vi "File Page - Update Multi-Trig Controls.vi"(7 "File Ctl Refs in":T2, 8 "error in (no error)":errorcluster, 11 "Item Ref in":T1 format="%.0x") -> (0 "error out":errorcluster)   [LabVIEW 2015, in "Waveform Data Logger System Explorer.lvlib"]
uses:
  Waveform Data Logger System Explorer.lvlib
  Types/File Ctl Refs.ctl
  Types/File - Spec Ctl Refs.ctl
  Types/File - Wfm Ctl Refs.ctl
  Types/File - Settings Ctl Refs.ctl
  Shared/Classes/Log File Specifications/Log File Specification/File Conflict Operation.ctl
  Types/File - Start Trig Ctl Refs.ctl
  Shared/Types/Start Trigger.ctl
  Shared/Types/Default Trigger.ctl
  Shared/Types/Digital Trigger.ctl
  Shared/Types/Analog Trigger.ctl
  Shared/Types/In Range Trigger.ctl
  Shared/Types/Value Change Trigger.ctl
  Shared/Types/Boolean Trigger.ctl
  Types/Single Node Browser Data.ctl
  <vilib>/NI Veristand/UI Controls/Single Node Browser/Single Node Browser Ref.ctl
  NationalInstruments.VeriStand.SystemStorageUI
  <vilib>/NI Veristand/UI Controls/Single Node Browser/Callback Type.ctl
  <vilib>/NI Veristand/UI Controls/Single Node Browser/Net Event Data.ctl
  <vilib>/NI Veristand/UI Controls/Single Node Browser/Net Event.ctl
  Types/File - Stop Trig Ctl Refs.ctl
  Shared/Types/Stop Trigger.ctl
  Types/File - Advanced Ctl Refs.ctl
  Types/Log Timestamps.ctl
  <vilib>/NI Veristand/Custom Device API/Custom Device Item Ref.ctl
  Shared/Globals/Property Strings.vi
  <vilib>/NI Veristand/Custom Device API/Get Item Property (U16).vi
  <vilib>/NI Veristand/Custom Device API/Set Item Property (Boolean).vi
  <vilib>/NI Veristand/Custom Device API/Get Item Property (Boolean).vi
  Shared/Waveform Data Logger Shared.lvlib
  <vilib>/NI VeriStand/Custom Device API/Custom Device API.lvlib
  Shared/Classes/Log File Specifications/Log File Specification/Log File Specification.lvclass
  <vilib>/NI VeriStand/UI Controls/Single Node Browser/NI_VS UI Single Node Browser.lvlib
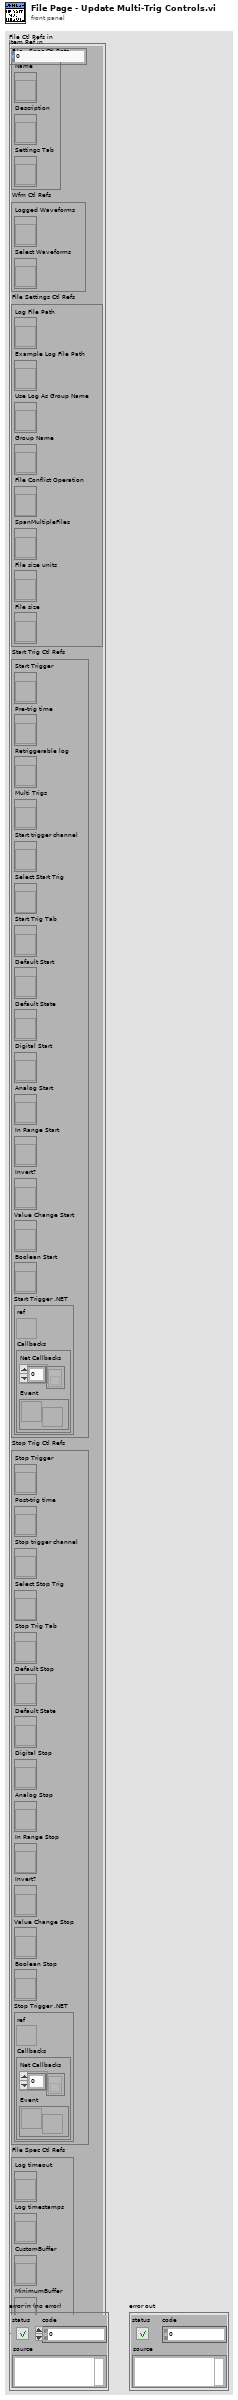
[diagram p1: front panel]
types:
  T1 = typedef "Custom Device API.lvlib/Custom Device Item Ref.ctl" = u64
  T2 = typedef "Waveform Data Logger System Explorer.lvlib/File Ctl Refs.ctl" = cluster{"File Spec Ctl Refs":T3, "Wfm Ctl Refs":T4, "File Settings Ctl Refs":T5, "Start Trig Ctl Refs":T6, "Stop Trig Ctl Refs":T10, "File Spec Ctl Refs":T11}
  T3 = typedef "Waveform Data Logger System Explorer.lvlib/File - Spec Ctl Refs.ctl" = cluster{"Name":refnum<vi>, "Description":refnum<vi>, "Settings Tab":refnum<vi>}
  T4 = typedef "Waveform Data Logger System Explorer.lvlib/File - Wfm Ctl Refs.ctl" = cluster{"Logged Waveforms":refnum<vi>, "Select Waveforms":refnum<vi>}
  T5 = typedef "Waveform Data Logger System Explorer.lvlib/File - Settings Ctl Refs.ctl" = cluster{"Log File Path":refnum<vi>, "Example Log File Path":refnum<vi>, "Use Log As Group Name":refnum<vi>, "Group Name":refnum<vi>, "File Conflict Operation":refnum<vi>, "SpanMultipleFiles":refnum<vi>, "File size units":refnum<vi>, "File size":refnum<vi>}
  T6 = typedef "Waveform Data Logger System Explorer.lvlib/File - Start Trig Ctl Refs.ctl" = cluster{"Start Trigger":refnum<vi>, "Pre-trig time":refnum<vi>, "Retriggerable log":refnum<vi>, "Multi Trigs":refnum<vi>, "Start trigger channel":refnum<vi>, "Select Start Trig":refnum<vi>, "Start Trig Tab":refnum<vi>, "Default Start":refnum<vi>, "Default State":refnum<vi>, "Digital Start":refnum<vi>, "Analog Start":refnum<vi>, "In Range Start":refnum<vi>, "Invert?":refnum<vi>, "Value Change Start":refnum<vi>, "Boolean Start":refnum<vi>, "Start Trigger .NET":T7}
  T7 = typedef "Waveform Data Logger System Explorer.lvlib/Single Node Browser Data.ctl" = cluster{"ref":T8, "Callbacks":T9}
  T8 = typedef "NI_VS UI Single Node Browser.lvlib/Single Node Browser Ref.ctl" = refnum<k24>
  T9 = typedef "NI_VS UI Single Node Browser.lvlib/Callback Type.ctl" = cluster{"Net Callbacks":refnum<k27>[], "Event":refnum<user-event>}
  T10 = typedef "Waveform Data Logger System Explorer.lvlib/File - Stop Trig Ctl Refs.ctl" = cluster{"Stop Trigger":refnum<vi>, "Post-trig time":refnum<vi>, "Stop trigger channel":refnum<vi>, "Select Stop Trig":refnum<vi>, "Stop Trig Tab":refnum<vi>, "Default Stop":refnum<vi>, "Default State":refnum<vi>, "Digital Stop":refnum<vi>, "Analog Stop":refnum<vi>, "In Range Stop":refnum<vi>, "Invert?":refnum<vi>, "Value Change Stop":refnum<vi>, "Boolean Stop":refnum<vi>, "Stop Trigger .NET":T7}
  T11 = typedef "Waveform Data Logger System Explorer.lvlib/File - Advanced Ctl Refs.ctl" = cluster{"Log timeout":refnum<vi>, "Log timestamps":refnum<vi>, "CustomBuffer":refnum<vi>, "MinimumBuffer":refnum<vi>}
  T12 = typedef "Waveform Data Logger Shared.lvlib/Start Trigger.ctl" = enum16{"Start immediately", "Start on digital edge", "Start on analog edge", "Start when in range", "Start when out of range", "Start on value change", "Start when Boolean condition is true"}
  T13 = enum8{"Enabled", "Disabled", "Disabled and Grayed Out"}
  T14 = typedef "Waveform Data Logger Shared.lvlib/Stop Trigger.ctl" = enum16{"Log indefinitely", "Stop after duration", "Stop on digital edge", "Stop on analog edge", "Stop when in range", "Stop when out of range", "Stop on value change", "Stop when Boolean condition is true"}
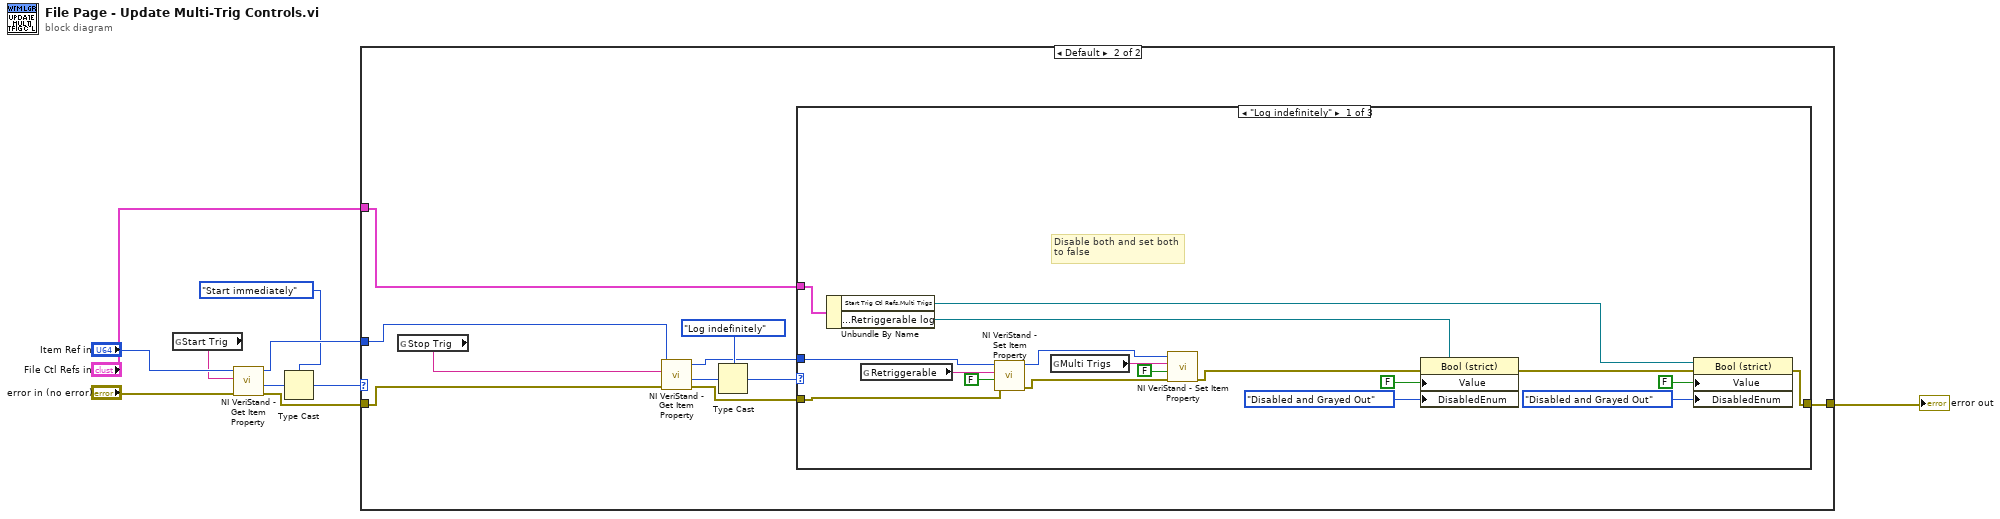
[diagram p0: block diagram]
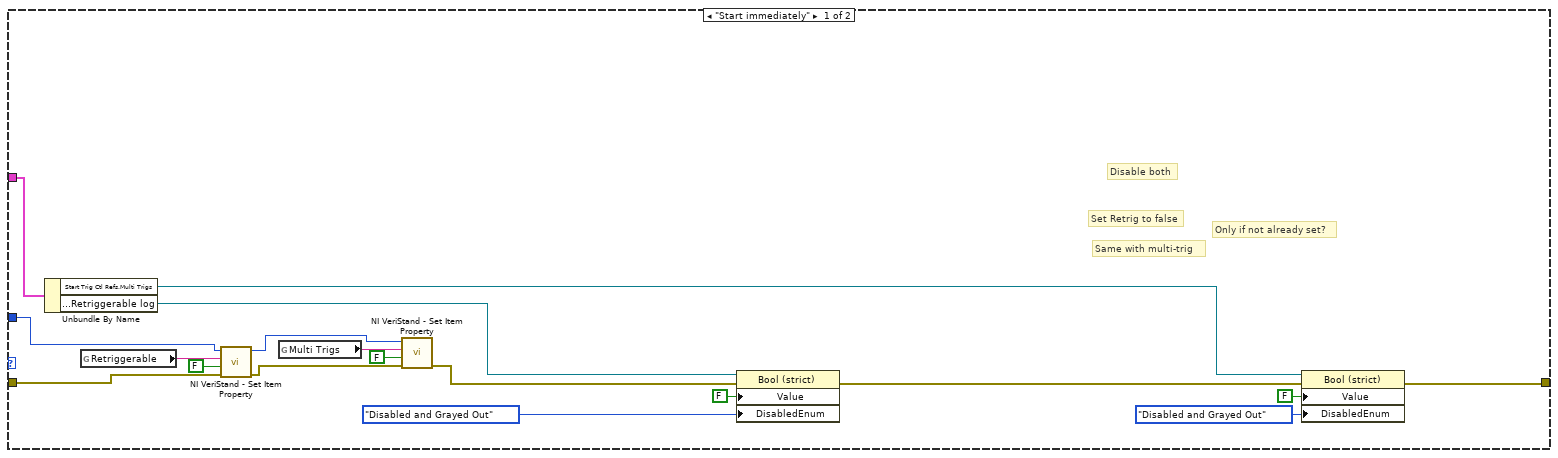
[diagram p2: hidden frame]
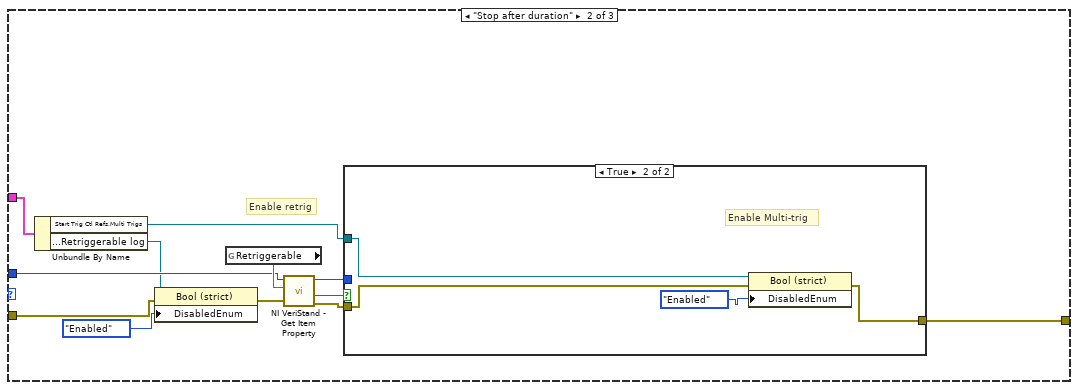
[diagram p3: hidden frame]
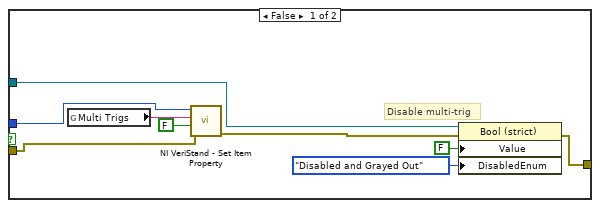
[diagram p4: hidden frame]
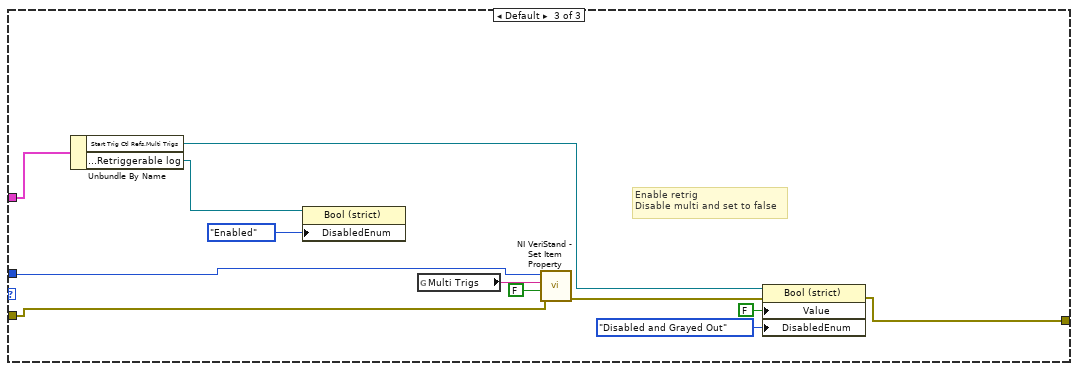
[diagram p5: hidden frame]
diagram:
  n1 = global read "Property Strings.vi" "Start Trig"() -> (w3:string)
  n2 = call-poly <vilib>:"NI VeriStand - Get Item Property.vi"("error in (no error)"="error in (no error)", "Property Name"=w3, "Item Ref in"="Item Ref in") -> ("error out"=w2:errorcluster, "Value"=w6:u16, "Item Ref out"=w10:T1)  [unwired: 1 in, 5 out]
  n3 = Type Cast(type=Start_Trigger."Start immediately" ("Start Trigger"), x=w6) -> (*(type *) &x=w8:T12)
  n4 = case shown="Default" w8 {
    tunnel: "File Ctl Refs in" -> [w28 w30]
    tunnel: w10 -> [w18 w33]
    tunnel: w2 -> [w17 w34]
    tunnel: [w20 w29] -> w1
    frame "Start immediately" {
      # "Only if not already set?"
      # "Same with multi-trig"
      # "Set Retrig to false"
      # "Disable both"
      n5 = Unbundle By Name(w28) -> ("Start Trig Ctl Refs.Multi Trigs"=w22:refnum<vi>, "Start Trig Ctl Refs.Retriggerable log"=w27:refnum<vi>)
      n6 = global read "Property Strings.vi" "Retriggerable"() -> (w19:string)
      n7 = call-poly <vilib>:"NI VeriStand - Set Item Property.vi"("error in (no error)"=w17, "Value"=FALSE, "Property Name"=w19, "Item Ref in"=w18) -> ("error out"=w14:errorcluster, "Item Ref out"=w13:T1)  [unwired: 5 in, 1 out]
      n8 = global read "Property Strings.vi" "Multi Trigs"() -> (w15:string)
      n9 = call-poly <vilib>:"NI VeriStand - Set Item Property.vi"("error in (no error)"=w14, "Value"=FALSE, "Property Name"=w15, "Item Ref in"=w13) -> ("error out"=w11:errorcluster)  [unwired: 5 in, 2 out]
      n10 = property class="Bool (strict)"(reference=w27, error in=w11, "Value"=FALSE, "DisabledEnum"=T13."Disabled and Grayed Out" ("Disabled")) -> (error out=w21:errorcluster)  [unwired: 1 out]
      n11 = property class="Bool (strict)"(reference=w22, error in=w21, "Value"=FALSE, "DisabledEnum"=T13."Disabled and Grayed Out" ("Disabled")) -> (error out=w20:errorcluster)  [unwired: 1 out]
    }
    frame Default {
      n12 = global read "Property Strings.vi" "Stop Trig"() -> (w38:string)
      n13 = call-poly <vilib>:"NI VeriStand - Get Item Property.vi"("error in (no error)"=w34, "Property Name"=w38, "Item Ref in"=w33) -> ("error out"=w32:errorcluster, "Value"=w37:u16, "Item Ref out"=w31:T1)  [unwired: 1 in, 5 out]
      n14 = Type Cast(type=Stop_Trigger."Log indefinitely" ("Stop Trigger"), x=w37) -> (*(type *) &x=w35:T14)
      n15 = case shown="\"Log indefinitely\"" w35 {
        tunnel: w32 -> [w40 w63 w87]
        tunnel: w31 -> [w39 w66 w88]
        tunnel: w30 -> [w41 w65 w93]
        tunnel: [w42 w58 w82] -> w29
        frame "Log indefinitely" {
          # "Disable both and set both\nto false"
          n16 = Unbundle By Name(w41) -> ("Start Trig Ctl Refs.Multi Trigs"=w51:refnum<vi>, "Start Trig Ctl Refs.Retriggerable log"=w56:refnum<vi>)
          n17 = global read "Property Strings.vi" "Retriggerable"() -> (w49:string)
          n18 = call-poly <vilib>:"NI VeriStand - Set Item Property.vi"("error in (no error)"=w40, "Value"=FALSE, "Property Name"=w49, "Item Ref in"=w39) -> ("error out"=w46:errorcluster, "Item Ref out"=w45:T1)  [unwired: 5 in, 1 out]
          n19 = global read "Property Strings.vi" "Multi Trigs"() -> (w47:string)
          n20 = call-poly <vilib>:"NI VeriStand - Set Item Property.vi"("error in (no error)"=w46, "Value"=FALSE, "Property Name"=w47, "Item Ref in"=w45) -> ("error out"=w43:errorcluster)  [unwired: 5 in, 2 out]
          n21 = property class="Bool (strict)"(reference=w56, error in=w43, "Value"=FALSE, "DisabledEnum"=T13."Disabled and Grayed Out" ("Disabled")) -> (error out=w50:errorcluster)  [unwired: 1 out]
          n22 = property class="Bool (strict)"(reference=w51, error in=w50, "Value"=FALSE, "DisabledEnum"=T13."Disabled and Grayed Out" ("Disabled")) -> (error out=w42:errorcluster)  [unwired: 1 out]
        }
        frame "Stop after duration" {
          # "Enable retrig"
          n23 = Unbundle By Name(w65) -> ("Start Trig Ctl Refs.Multi Trigs"=w60:refnum<vi>, "Start Trig Ctl Refs.Retriggerable log"=w64:refnum<vi>)
          n24 = property class="Bool (strict)"(reference=w64, error in=w63, "DisabledEnum"=T13."Enabled" ("Disabled")) -> (error out=w61:errorcluster)  [unwired: 1 out]
          n25 = global read "Property Strings.vi" "Retriggerable"() -> (w68:string)
          n26 = call-poly <vilib>:"NI VeriStand - Get Item Property.vi"("error in (no error)"=w61, "Property Name"=w68, "Item Ref in"=w66) -> ("error out"=w59:errorcluster, "Value"=w67:bool, "Item Ref out"=w57:T1)  [unwired: 1 in, 5 out]
          n27 = case shown="True" w67 {
            tunnel: w60 -> [w71 w81]
            tunnel: w59 -> [w70 w79]
            tunnel: [w75 w78] -> w58
            tunnel: w57 -> [w72 _]
            frame False {
              # "Disable multi-trig"
              n28 = global read "Property Strings.vi" "Multi Trigs"() -> (w74:string)
              n29 = call-poly <vilib>:"NI VeriStand - Set Item Property.vi"("error in (no error)"=w70, "Value"=FALSE, "Property Name"=w74, "Item Ref in"=w72) -> ("error out"=w69:errorcluster)  [unwired: 5 in, 2 out]
              n30 = property class="Bool (strict)"(reference=w71, error in=w69, "Value"=FALSE, "DisabledEnum"=T13."Disabled and Grayed Out" ("Disabled")) -> (error out=w75:errorcluster)  [unwired: 1 out]
            }
            frame True {
              # "Enable Multi-trig"
              n31 = property class="Bool (strict)"(reference=w81, error in=w79, "DisabledEnum"=T13."Enabled" ("Disabled")) -> (error out=w78:errorcluster)  [unwired: 1 out]
            }
          }
        }
        frame Default {
          # "Enable retrig\nDisable multi and set to false"
          n32 = Unbundle By Name(w93) -> ("Start Trig Ctl Refs.Multi Trigs"=w83:refnum<vi>, "Start Trig Ctl Refs.Retriggerable log"=w91:refnum<vi>)
          n33 = property class="Bool (strict)"(reference=w91, "DisabledEnum"=T13."Enabled" ("Disabled")) -> ()  [unwired: 1 in, 2 out]
          n34 = global read "Property Strings.vi" "Multi Trigs"() -> (w90:string)
          n35 = call-poly <vilib>:"NI VeriStand - Set Item Property.vi"("error in (no error)"=w87, "Value"=FALSE, "Property Name"=w90, "Item Ref in"=w88) -> ("error out"=w84:errorcluster)  [unwired: 5 in, 2 out]
          n36 = property class="Bool (strict)"(reference=w83, error in=w84, "Value"=FALSE, "DisabledEnum"=T13."Disabled and Grayed Out" ("Disabled")) -> (error out=w82:errorcluster)  [unwired: 1 out]
        }
      }
    }
  }
  "error out" <- w1
